vi "hot_plate_control_subVI.vi"(2 "LoadCell":u32, 3 "Stop-button":bool, 4 "Array":dbl[](array[numeric])) -> (0 "Numeric":dbl, 1 "Warmer\nON":bool)   [LabVIEW 2021]
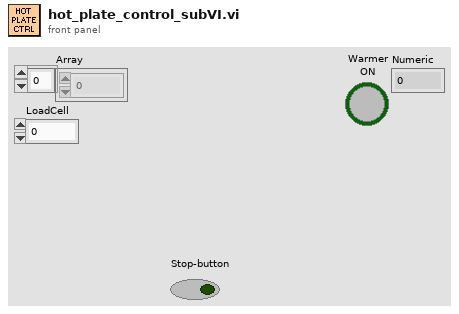
[diagram p1: front panel]
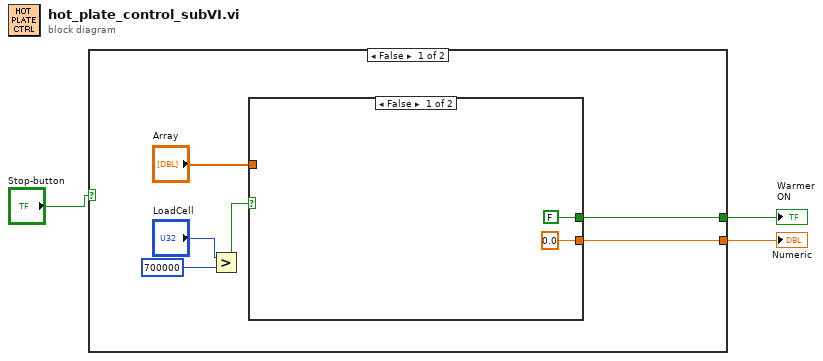
[diagram p0: block diagram]
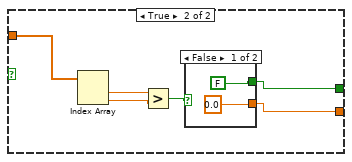
[diagram p2: hidden frame]
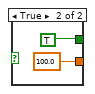
[diagram p3: hidden frame]
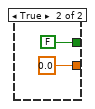
[diagram p4: hidden frame]
diagram:
  n1 = case shown="False" "Stop-button" {
    tunnel: [w5 0.0] -> w2
    tunnel: [w4 FALSE] -> w1
    frame False {
      n2 = Greater?(x="LoadCell", y=u32 700000) -> (0:w6:bool)
      n3 = case shown="False" w6 {
        tunnel: "Array" -> [_ w17]
        tunnel: [0.0 w13] -> w5
        tunnel: [FALSE w12] -> w4
        frame False {
        }
        frame True {
          n4 = Index Array(array=w17) -> (element #1=w16:dbl, element #2=w15:dbl)  [unwired: 2 in]
          n5 = Greater?(x=w16, y=w15) -> (0:w14:bool)
          n6 = case shown="False" w14 {
            tunnel: [FALSE TRUE] -> w12
            tunnel: [0.0 100.0] -> w13
            frame False {
            }
            frame True {
            }
          }
        }
      }
    }
    frame True {
    }
  }
  "Warmer\nON" <- w1
  "Numeric" <- w2
